vi "Time_Transform.vi"(0 "Elapsed Time (s)":dbl) -> (1 "Temps Total":string)   [LabVIEW 2017]
panel:
  out "concatenated string":string
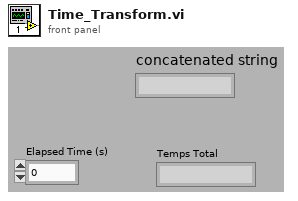
[diagram p1: front panel]
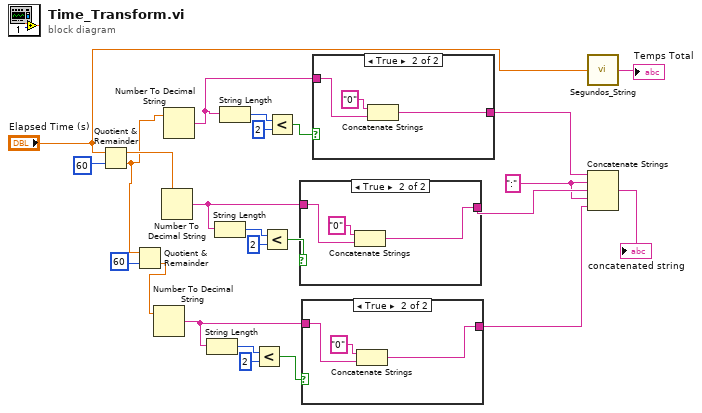
[diagram p0: block diagram]
diagram:
  w10 = ":" ("string")
  n1 = Quotient & Remainder(x="Elapsed Time (s)", y=u16 60) -> (x-y*floor(x/y)=w24:dbl, floor(x/y)=w22:dbl)
  n2 = Quotient & Remainder(x=w22, y=u16 60) -> (floor(x/y)=w4:dbl)  [unwired: 1 out]
  n3 = Number To Decimal String(number=w4) -> (decimal integer string=w7:string)  [unwired: 1 in]
  n4 = Number To Decimal String(number=w24) -> (decimal integer string=w17:string)  [unwired: 1 in]
  n5 = Number To Decimal String(number=w22) -> (decimal integer string=w12:string)  [unwired: 1 in]
  n6 = String Length(string=w7) -> (length=w9:i32)
  n7 = String Length(string=w17) -> (length=w20:i32)
  n8 = String Length(string=w12) -> (length=w14:i32)
  n9 = Less?(x=w9, y=2) -> (x < y?=w6:bool)
  n10 = Less?(x=w20, y=2) -> (x < y?=w18:bool)
  n11 = Less?(x=w14, y=2) -> (x < y?=w11:bool)
  n12 = case shown="True" w18 {
    tunnel: w17 -> [w25 w27]
    tunnel: [w25 w26] -> w16
    frame False {
    }
    frame True {
      n13 = Concatenate Strings("0" ("string"), w27) -> (w26:string)
    }
  }
  n14 = case shown="True" w6 {
    tunnel: w7 -> [w29 w31]
    tunnel: [w29 w30] -> w5
    frame False {
    }
    frame True {
      n15 = Concatenate Strings("0" ("string"), w31) -> (w30:string)
    }
  }
  n16 = case shown="True" w11 {
    tunnel: w12 -> [w33 w35]
    tunnel: [w33 w34] -> w15
    frame False {
    }
    frame True {
      n17 = Concatenate Strings("0" ("string"), w35) -> (w34:string)
    }
  }
  n18 = call "Segundos_String.vi"("Total sec"="Elapsed Time (s)") -> ("TempsTotal"=→"Temps Total":string)
  n19 = Concatenate Strings(w15, w10, w16, w10, w5) -> (→"concatenated string":string)
